vi "Set Multi Track H Range.vi"(8 "error in (no error)":errorcluster, 10 "iEnd":i32, 11 "iStart":i32) -> (0 "error out":errorcluster, 3 "function return":u32)   [LabVIEW 2014, in "atmcd32d.lvlib"]
doc: "unsigned int WINAPI SetMultiTrackHRange(int iStart, int iEnd);"
uses:
  atmcd32d.lvlib
  atmcd32d.dll
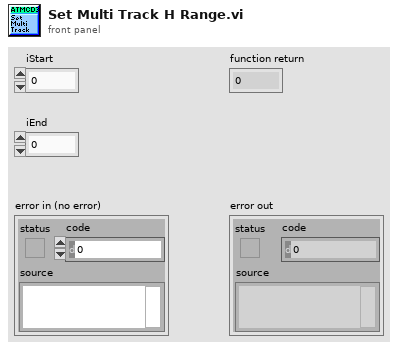
[diagram p1: front panel]
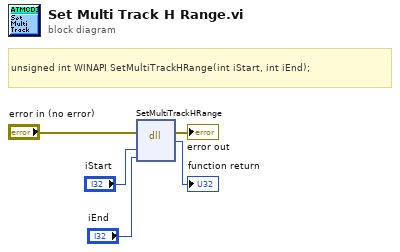
[diagram p0: block diagram]
diagram:
  # "unsigned int WINAPI SetMultiTrackHRange(int iStart, int iEnd);"
  n1 = dll-call lib="C:/Users/Bakir/Documents/Lambda2-Testing/lib/Andorlib/atmcd32d.*" fn="SetMultiTrackHRange"(error in="error in (no error)", "iStart"="iStart", "iEnd"="iEnd") -> (error out=→"error out":errorcluster, →"function return":u32)  [unwired: 4 in, 1 out]
